vi "Fick to Rotation Matrix.vi"(1 "T":dbl format="%.2f", 2 "V":dbl format="%.2f", 3 "H":dbl format="%.2f") -> (0 "Rotation Matrix":dbl[][](array[numeric]) format="%.2f")   [LabVIEW 2016, in "fick-matrix.lvlib"]
uses:
  fick-matrix.lvlib
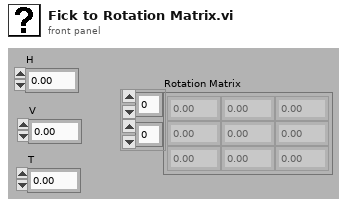
[diagram p1: front panel]
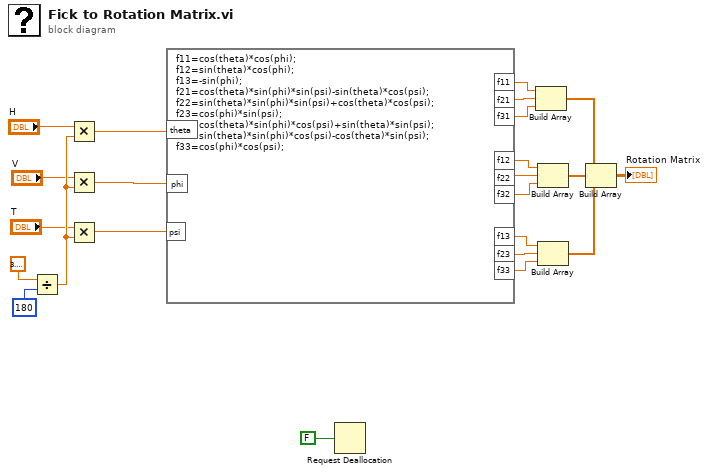
[diagram p0: block diagram]
diagram:
  n1 = Divide(x=3.141592653589793, y=180) -> (x/y=w21:dbl)
  n2 = Multiply(x="H", y=w21) -> (x*y=w17:dbl)
  n3 = Multiply(x="V", y=w21) -> (x*y=w16:dbl)
  n4 = Multiply(x="T", y=w21) -> (x*y=w15:dbl)
  n5 = formula code="f11=cos(theta)*cos(phi);\nf12=sin(theta)*cos(phi);\nf13=-sin(phi);\nf21=cos(theta)*sin(phi)*sin(psi)-sin(theta)*cos(psi);\nf22=sin(theta)*sin(phi)*sin(psi)+cos(theta)*cos(psi);\nf23=cos(phi)*sin(psi);\nf31=cos(theta)*sin(phi)*cos(psi)+sin(theta)*sin(psi);\nf32=sin(theta)*sin(phi)*cos(psi)-cos(theta)*sin(psi);\nf33=cos(phi)*cos(psi);"("theta"=w17, "phi"=w16, "psi"=w15) -> ("f11"=w14:dbl, "f21"=w13:dbl, "f31"=w12:dbl, "f22"=w9:dbl, "f23"=w7:dbl, "f12"=w11:dbl, "f32"=w10:dbl, "f13"=w8:dbl, "f33"=w6:dbl)
  n6 = Request Deallocation(FALSE ("flag")) -> ()
  n7 = Build Array(w14, w13, w12) -> (w5:dbl[])
  n8 = Build Array(w11, w9, w10) -> (w4:dbl[])
  n9 = Build Array(w8, w7, w6) -> (w3:dbl[])
  n10 = Build Array(w5, w4, w3) -> (→"Rotation Matrix":dbl[][])
